vi "SelectSignalPortion.vi"(1 "Column Indx":i32, 2 "length":i32, 3 "Start":i32, 4 "2D Array":dbl[][](array[numeric])) -> (0 "subarray":dbl[](array[numeric]))   [LabVIEW 2019]
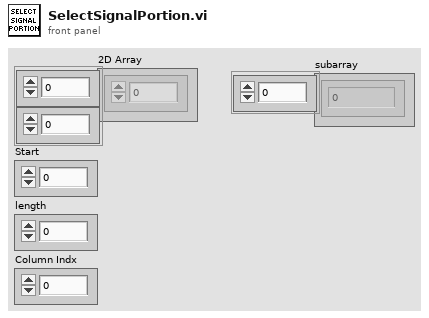
[diagram p1: front panel]
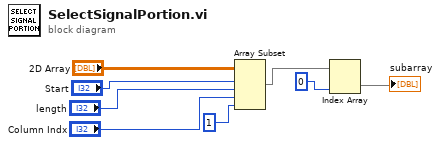
[diagram p0: block diagram]
diagram:
  n1 = Array Subset(array="2D Array", index (row)="Start", length (row)="length", index (col)="Column Indx", length (col)=1 ("length")) -> (w8:dbl[][])
  n2 = Index Array(array=w8, index (col)=0 ("index (row)")) -> (element=→"subarray":dbl[])  [unwired: 1 in]
